vi "mouseZoom.vi"(6 "XY":cluster{"X":dbl, "Y":dbl}, 8 "error in (no error)":errorcluster, 9 "Delta":i32, 10 "PlatMods":T1, 11 "QControl_Graph in":refnum<class "QControl_Graph.lvclass">) -> (0 "error out":errorcluster, 3 "QControl_Graph out":refnum<class "QControl_Graph.lvclass">)   [LabVIEW 2017, in "QControl_Graph.lvclass"]
uses:
  QControl_Graph.lvclass
  Actions.ctl
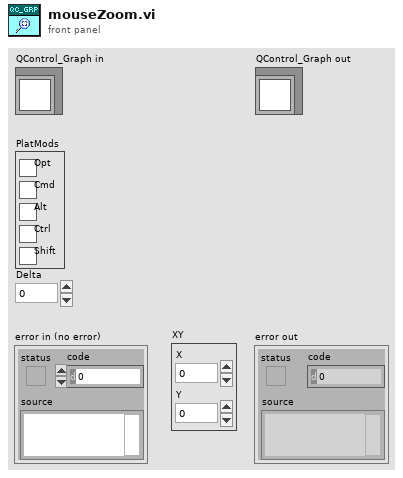
[diagram p1: front panel]
types:
  T1 = cluster{"Opt":bool, "Cmd":bool, "Alt":bool, "Ctrl":bool, "Shift":bool}
  T2 = typedef "QControl_Graph.lvclass/Actions.ctl" = enum16{"Undefined", "BGK Color", "Highlight Plot", "Mouse Zoom", "Show Cursors", "Cursor Properties", "Show Markers"}
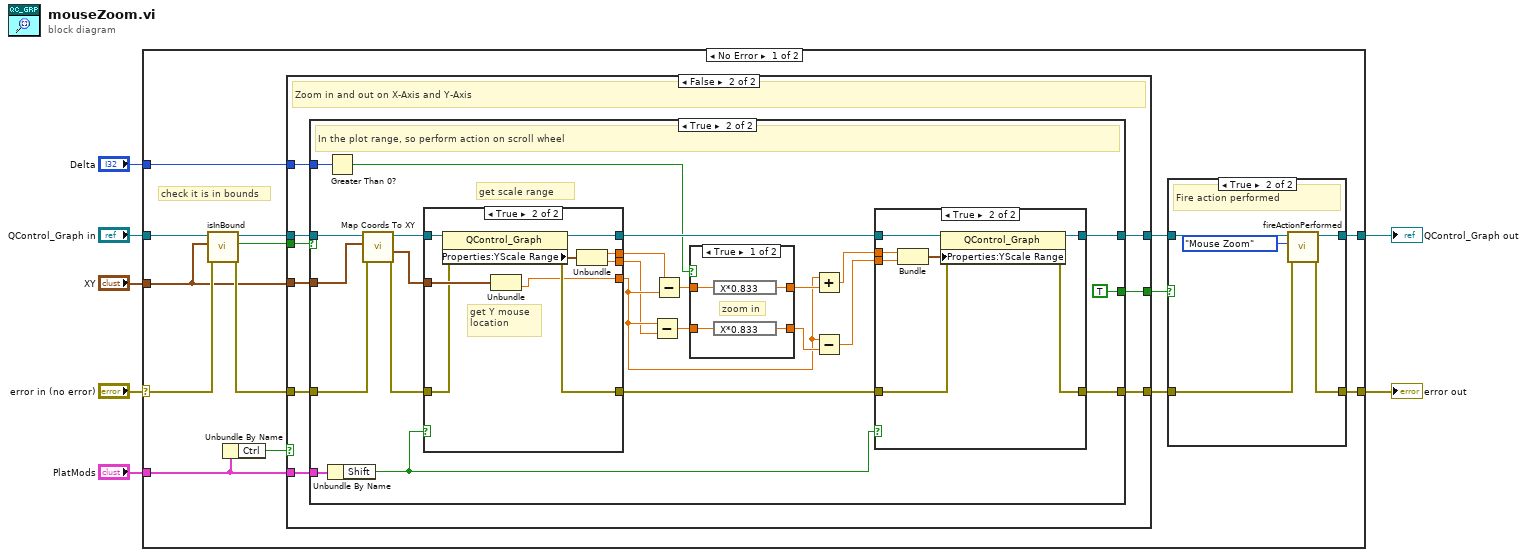
[diagram p0: block diagram]
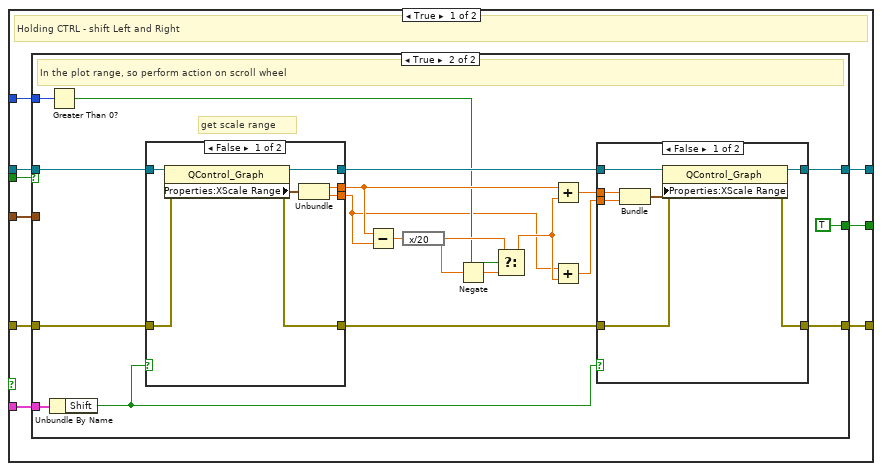
[diagram p3: hidden frame]
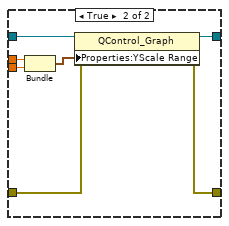
[diagram p5: hidden frame]
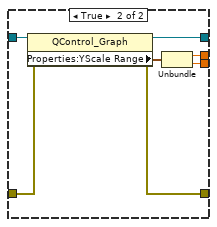
[diagram p6: hidden frame]
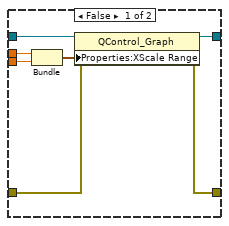
[diagram p8: hidden frame]
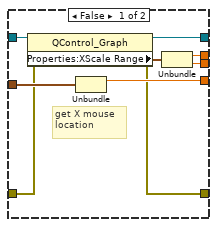
[diagram p9: hidden frame]
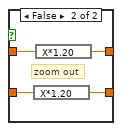
[diagram p10: hidden frame]
diagram:
  n1 = case shown="No Error" "error in (no error)" {
    tunnel: "XY" -> [w13 _]
    selector: "error in (no error)" -> [w15 w163]
    tunnel: [w11 w163] -> w6
    tunnel: [w9 w162] -> w4
    tunnel: "QControl_Graph in" -> [w14 w162]
    tunnel: "Delta" -> [w18 _]
    tunnel: "PlatMods" -> [w19 _]
    frame No Error {
      # "check it is in bounds"
      n2 = call "isInBound.vi"("error in (no error)"=w15, "XY"=w13, "QControl_Graph in"=w14) -> ("error out"=w16:errorcluster, "Boolean"=w21:bool, "QControl_Graph out"=w17:refnum<class "QControl_Graph.lvclass">)  [unwired: 6 in]
      n3 = Unbundle By Name(w19) -> ("Ctrl"=w20:bool)
      n4 = case shown="False" w20 {
        tunnel: w13 -> [w30 w88]
        tunnel: w21 -> [w37 w95]
        tunnel: w19 -> [w36 w94]
        tunnel: w18 -> [w35 w93]
        tunnel: w16 -> [w34 w92]
        tunnel: w17 -> [w33 w91]
        tunnel: [w32 w90] -> w12
        tunnel: [w31 w89] -> w10
        tunnel: [w29 w87] -> w8
        frame True {
          # "Holding CTRL - shift Left and Right"
          n5 = case shown="True" w37 {
            tunnel: w30 -> [_ _]
            tunnel: w35 -> [_ w56]
            tunnel: w33 -> [w38 w51]
            tunnel: w34 -> [w39 w50]
            tunnel: w36 -> [_ w55]
            tunnel: [w39 w53] -> w32
            tunnel: [w38 w52] -> w31
            tunnel: [_ TRUE] -> w29
            frame False {
              # "Not in the plot range, so ignore the scroll wheel"
            }
            frame True {
              # "get scale range"
              # "In the plot range, so perform action on scroll wheel"
              n6 = Greater Than 0?(x=w56) -> (x > 0?=w44:bool)
              n7 = Unbundle By Name(w55) -> ("Shift"=w54:bool)
              n8 = case shown="False" w54 {
                tunnel: [w74 w81] -> w45
                tunnel: [w73 w80] -> w41
                tunnel: [w79 w86] -> w58
                tunnel: [w78 w85] -> w57
                tunnel: w50 -> [w77 w84]
                tunnel: w51 -> [w76 w83]
                frame False {
                  n9 = property on="Property Node" class="QControl_Graph"(reference=w76, error in=w77) -> (reference out=w78:refnum<class "QControl_Graph.lvclass">, error out=w79:errorcluster, "Properties:XScale Range"=w75:cluster{"Maximum":dbl, "Minimum":dbl})
                  n10 = Unbundle(w75) -> ("Maximum"=w74:dbl, "Minimum"=w73:dbl)
                }
                frame True {
                  n11 = property on="Property Node" class="QControl_Graph"(reference=w83, error in=w84) -> (reference out=w85:refnum<class "QControl_Graph.lvclass">, error out=w86:errorcluster, "Properties:YScale Range"=w82:cluster{"Maximum":dbl, "Minimum":dbl})
                  n12 = Unbundle(w82) -> ("Maximum"=w81:dbl, "Minimum"=w80:dbl)
                }
              }
              n13 = Subtract(x=w45, y=w41) -> (x-y=w49:dbl)
              n14 = expression code="x/20"(w49) -> (w46:dbl)
              n15 = Negate(x=w46) -> (-x=w48:dbl)
              n16 = Select(t=w46, s=w44, f=w48) -> (s? t:f=w47:dbl)
              n17 = Add(x=w45, y=w47) -> (x+y=w43:dbl)
              n18 = Add(x=w41, y=w47) -> (x+y=w42:dbl)
              n19 = case shown="False" w54 {
                tunnel: w42 -> [w60 w67]
                tunnel: w43 -> [w61 w68]
                tunnel: w58 -> [w64 w71]
                tunnel: w57 -> [w65 w72]
                tunnel: [w63 w70] -> w52
                tunnel: [w62 w69] -> w53
                frame False {
                  n20 = Bundle(w61, w60) -> (w59:cluster{dbl, dbl})  [unwired: 1 in]
                  n21 = property on="Property Node" class="QControl_Graph"(reference=w65, error in=w64, "Properties:XScale Range"=w59) -> (reference out=w63:refnum<class "QControl_Graph.lvclass">, error out=w62:errorcluster)
                }
                frame True {
                  n22 = Bundle(w68, w67) -> (w66:cluster{dbl, dbl})  [unwired: 1 in]
                  n23 = property on="Property Node" class="QControl_Graph"(reference=w72, error in=w71, "Properties:YScale Range"=w66) -> (reference out=w70:refnum<class "QControl_Graph.lvclass">, error out=w69:errorcluster)
                }
              }
            }
          }
        }
        frame False {
          # "Zoom in and out on X-Axis and Y-Axis"
          n24 = case shown="True" w95 {
            tunnel: w88 -> [_ w105]
            tunnel: w93 -> [_ w117]
            tunnel: w91 -> [w96 w106]
            tunnel: w92 -> [w97 w104]
            tunnel: w94 -> [_ w115]
            tunnel: [w97 w101] -> w90
            tunnel: [w96 w100] -> w89
            tunnel: [_ TRUE] -> w87
            frame False {
              # "Not in the plot range, so ignore the scroll wheel"
            }
            frame True {
              # "get scale range"
              # "In the plot range, so perform action on scroll wheel"
              n25 = Greater Than 0?(x=w117) -> (x > 0?=w116:bool)
              n26 = Unbundle By Name(w115) -> ("Shift"=w114:bool)
              n27 = call-dynamic "Map Coords To XY.vi"("error in (no error)"=w104, "Coords"=w105, "GraphChart in"=w106) -> ("error out"=w103:errorcluster, "XY"=w98:cluster{"X":dbl, "Y":dbl}, "GraphChart out"=w102:refnum<class "QControl_Graph.lvclass">)  [unwired: 5 in, 1 out]
              n28 = case shown="True" w114 {
                tunnel: [w137 w147] -> w111
                tunnel: [w136 w146] -> w108
                tunnel: [w144 w145] -> w109
                tunnel: [w143 w153] -> w119
                tunnel: [w142 w152] -> w118
                tunnel: w98 -> [w141 w151]
                tunnel: w103 -> [w140 w150]
                tunnel: w102 -> [w139 w149]
                frame False {
                  # "get X mouse location"
                  n29 = property on="Property Node" class="QControl_Graph"(reference=w139, error in=w140) -> (reference out=w142:refnum<class "QControl_Graph.lvclass">, error out=w143:errorcluster, "Properties:XScale Range"=w138:cluster{"Maximum":dbl, "Minimum":dbl})
                  n30 = Unbundle(w141) -> ("X"=w144:dbl)  [unwired: 1 out]
                  n31 = Unbundle(w138) -> ("Maximum"=w137:dbl, "Minimum"=w136:dbl)
                }
                frame True {
                  # "get Y mouse location"
                  n32 = property on="Property Node" class="QControl_Graph"(reference=w149, error in=w150) -> (reference out=w152:refnum<class "QControl_Graph.lvclass">, error out=w153:errorcluster, "Properties:YScale Range"=w148:cluster{"Maximum":dbl, "Minimum":dbl})
                  n33 = Unbundle(w151) -> ("Y"=w145:dbl)  [unwired: 1 out]
                  n34 = Unbundle(w148) -> ("Maximum"=w147:dbl, "Minimum"=w146:dbl)
                }
              }
              n35 = Subtract(x=w109, y=w108) -> (x-y=w107:dbl)
              n36 = Subtract(x=w111, y=w109) -> (x-y=w110:dbl)
              n37 = case shown="True" w116 {
                tunnel: w110 -> [w157 w161]
                tunnel: [w156 w160] -> w120
                tunnel: w107 -> [w155 w159]
                tunnel: [w154 w158] -> w113
                frame True {
                  # "zoom in"
                  n38 = expression code="X*0.833"(w157) -> (w156:dbl)
                  n39 = expression code="X*0.833"(w155) -> (w154:dbl)
                }
                frame False {
                  # "zoom out"
                  n40 = expression code="X*1.20"(w159) -> (w158:dbl)
                  n41 = expression code="X*1.20"(w161) -> (w160:dbl)
                }
              }
              n42 = Add(x=w109, y=w120) -> (x+y=w121:dbl)
              n43 = Subtract(x=w109, y=w113) -> (x-y=w112:dbl)
              n44 = case shown="True" w114 {
                tunnel: w112 -> [w123 w130]
                tunnel: w121 -> [w124 w131]
                tunnel: w119 -> [w127 w134]
                tunnel: w118 -> [w128 w135]
                tunnel: [w126 w133] -> w100
                tunnel: [w125 w132] -> w101
                frame False {
                  n45 = Bundle(w124, w123) -> (w122:cluster{dbl, dbl})  [unwired: 1 in]
                  n46 = property on="Property Node" class="QControl_Graph"(reference=w128, error in=w127, "Properties:XScale Range"=w122) -> (reference out=w126:refnum<class "QControl_Graph.lvclass">, error out=w125:errorcluster)
                }
                frame True {
                  n47 = Bundle(w131, w130) -> (w129:cluster{dbl, dbl})  [unwired: 1 in]
                  n48 = property on="Property Node" class="QControl_Graph"(reference=w135, error in=w134, "Properties:YScale Range"=w129) -> (reference out=w133:refnum<class "QControl_Graph.lvclass">, error out=w132:errorcluster)
                }
              }
            }
          }
        }
      }
      n49 = case shown="True" w8 {
        tunnel: w12 -> [w23 w26]
        tunnel: [w23 w25] -> w11
        tunnel: w10 -> [w22 w28]
        tunnel: [w22 w27] -> w9
        frame False {
          # "No action done"
        }
        frame True {
          # "Fire action performed"
          n50 = call-dynamic "fireActionPerformed.vi"("error in (no error)"=w26, "Action"=Actions."Mouse Zoom", "QControl_Graph in"=w28) -> ("error out"=w25:errorcluster, "QControl_Graph out"=w27:refnum<class "QControl_Graph.lvclass">)  [unwired: 7 in]
        }
      }
    }
    frame Error {
    }
  }
  "error out" <- w6
  "QControl_Graph out" <- w4
